vi "EOL_ITECHData.vi"(8 "Exit Program":refnum<vi>, 9 "PS Voltage":dbl=13.5, 10 "idx":u16, 11 "VISA name":refnum<visa-resource-name>) -> ()   [LabVIEW 2018]
uses:
  ZUP_Current/Def Ctrl/TestSeq.ctl
  ZUP_Current/Data buffer/ST0 current buffer.vi
  ZUP_Current/Data buffer/ST1 current buffer.vi
  ZUP_Current/Data buffer/ST2 current buffer.vi
  ZUP_Current/Data buffer/ST3 current buffer.vi
  ZUP_Current/Data buffer/ST4 current buffer.vi
  ZUP_Current/Data buffer/ST5 current buffer.vi
  05.UserVI's/Lambda Power/ITECH/IT-M3100.lvlib
panel:
  in  "Serial Configuration":T1={"Baud Rate"=9600, "Parity"=0, "Data Bits"=8, "Stop Bits"=10} {"Stop Bits" items=["1.0"=10, "1.5"=15, "2.0"=20]; "Data Bits" items=["7"=7, "8"=8]; "Parity" items=["None", "Odd", "Even", "Mark", "Space"]; "Baud Rate" items=["300"=300, "600"=600, "1200"=1200, "2400"=2400, "4800"=4800, "9600"=9600, "19200"=19200]}
  out "Max Cur":dbl
  out "Cur":dbl
  out "loss?":bool
  out "Packet loss":i32
  out "current":dbl(graph)
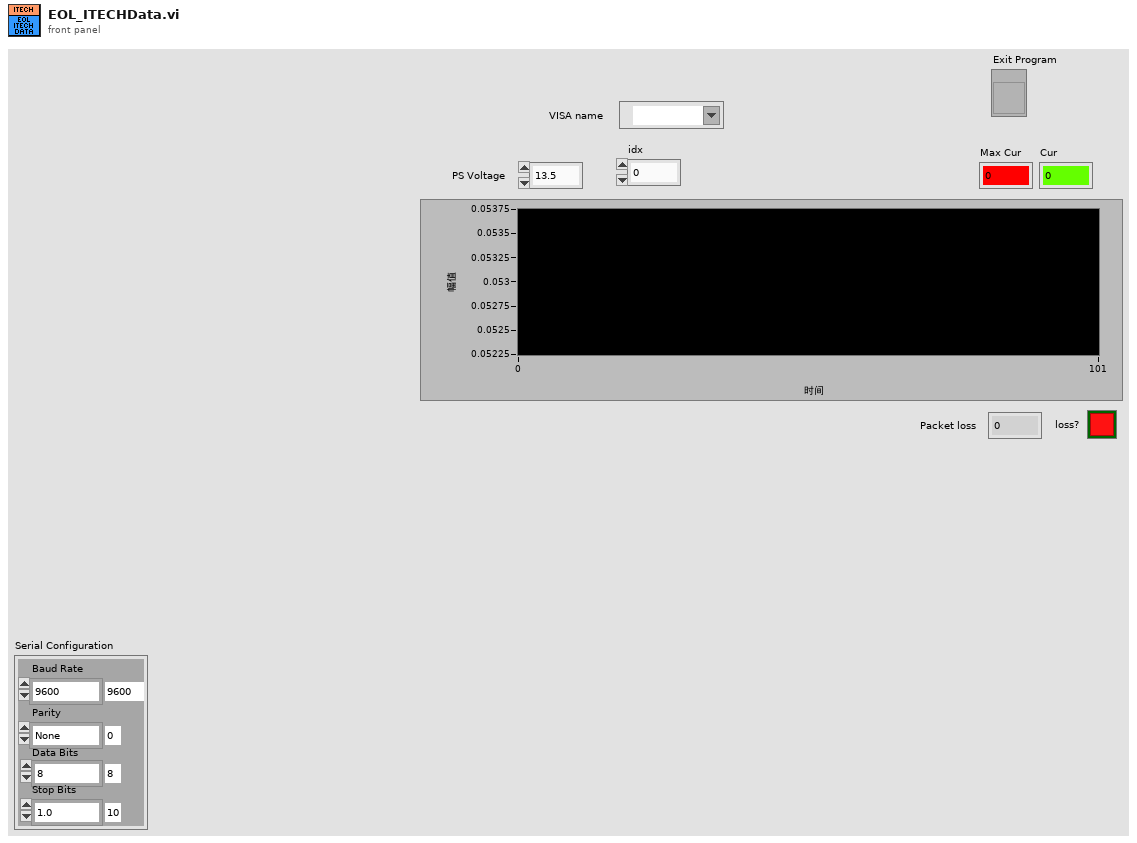
[diagram p1: front panel]
types:
  T1 = cluster{"Baud Rate":u32, "Parity":u16, "Data Bits":u16, "Stop Bits":u16}
  T2 = typedef "TestSeq.ctl" = enum16{"Idle", "Re Connect", "Error", "Initial", "Set Voltage", "Set Current", "Set Out", "Check Voltage", "Check Current", "Check Version No", "Check Out", "Get Current Data", "EOL Get Current Data"}
  T3 = cluster{"Serial Configuration":cluster{"Baud Rate":u32, "Parity":u16, "Data Bits":u16, "Stop Bits":u16}, "VISA name":refnum<visa-resource-name>, "MsgRec":string, "Current buffer":dbl[], "Timer":i32, "CycleNumb":i32, "Error":errorcluster, "Max Cur":dbl, "PS Voltage":dbl}
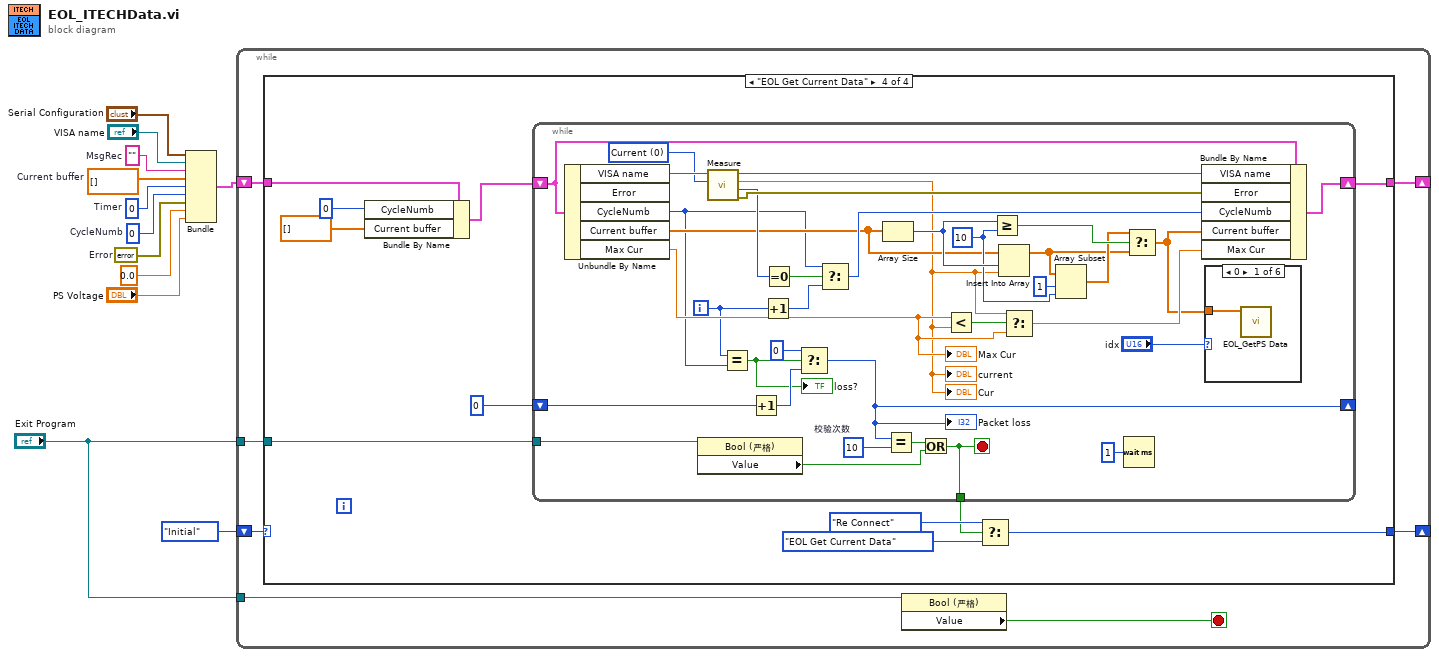
[diagram p0: block diagram]
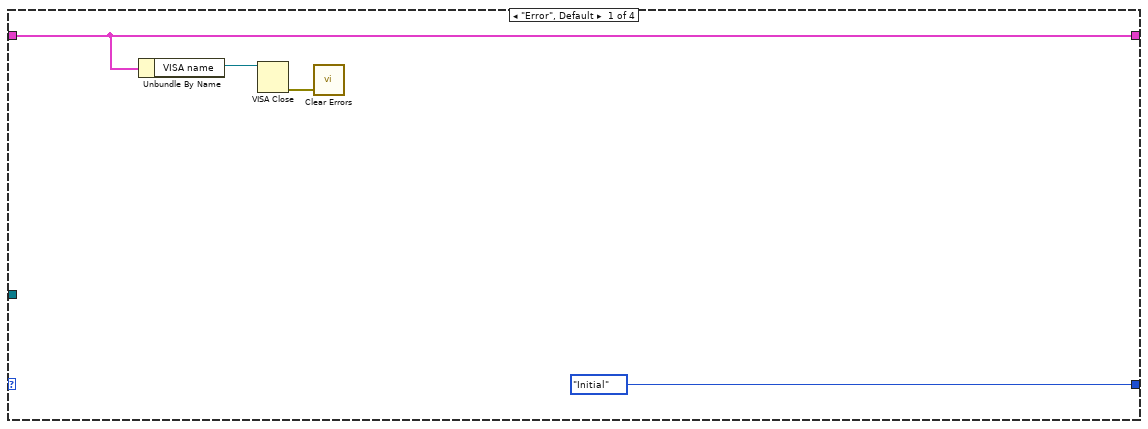
[diagram p2: hidden frame]
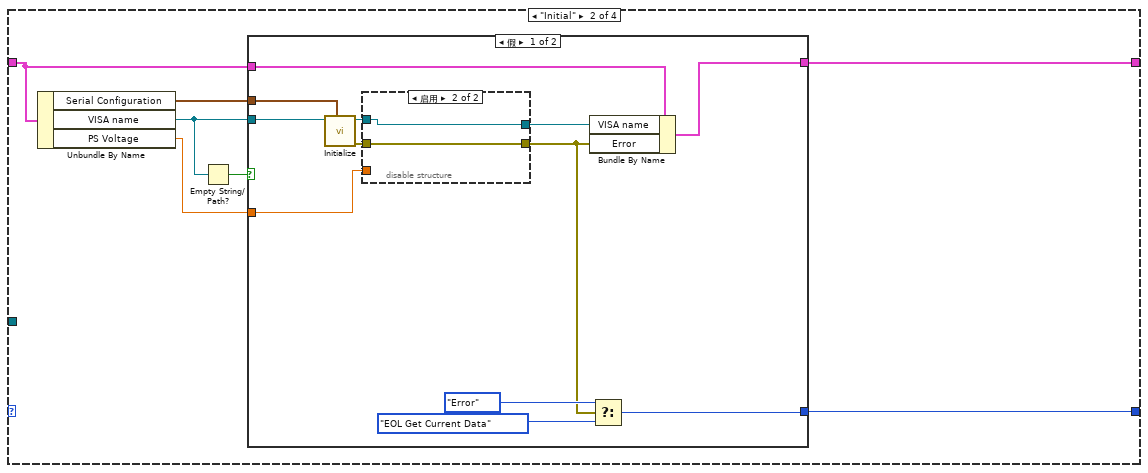
[diagram p3: hidden frame]
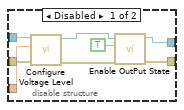
[diagram p4: hidden frame]
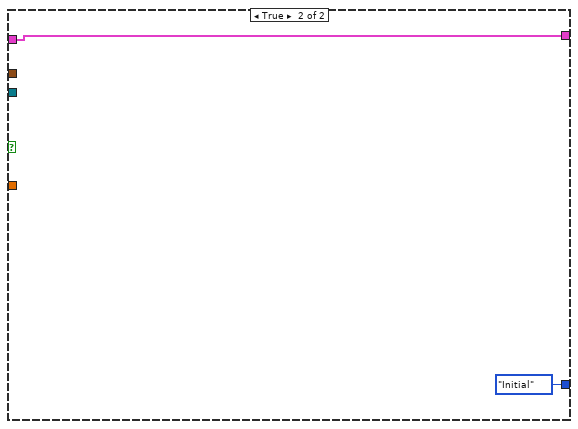
[diagram p5: hidden frame]
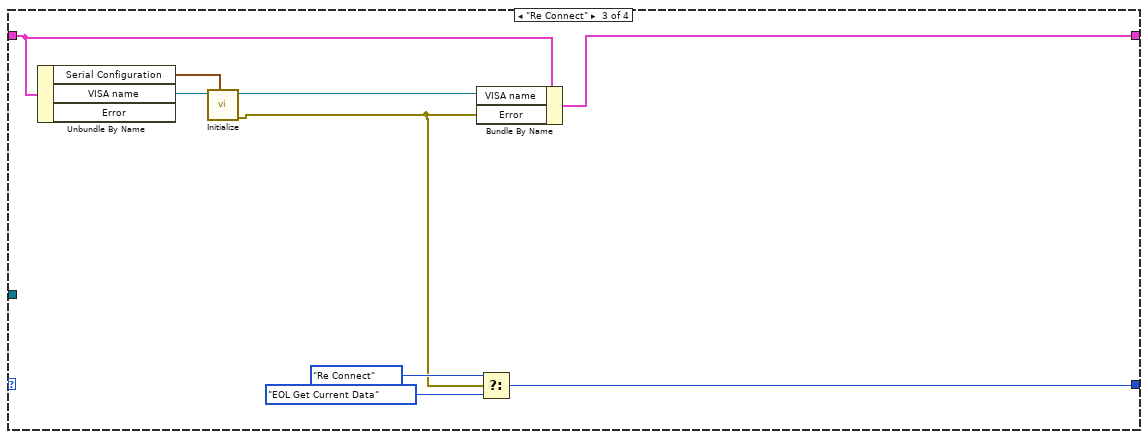
[diagram p6: hidden frame]
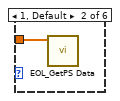
[diagram p7: hidden frame]
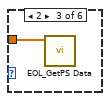
[diagram p8: hidden frame]
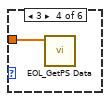
[diagram p9: hidden frame]
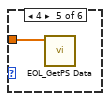
[diagram p10: hidden frame]
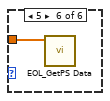
[diagram p11: hidden frame]
diagram:
  w5 = errorcluster {"status"=FALSE, "code"=0, "source"=""}  # Error
  w8 = 0  # CycleNumb
  w9 = 0  # Timer
  w12 = ""  # MsgRec
  w11 = dbl[] []  # Current buffer
  n1 = Bundle("Serial Configuration"="Serial Configuration", "VISA name"="VISA name", "MsgRec"=w12, "Current buffer"=w11, "Timer"=w9, "CycleNumb"=w8, "Error"=w5, "Max Cur"=0.0, "PS Voltage"="PS Voltage") -> (w7:T3)  [unwired: 1 in]
  n2 = while {
    shift-right: [w17] -> _
    shift-left: w7 -> [w18]
    shift-right: [w16] -> _
    shift-left: TestSeq."Initial" -> [w19]
    tunnel: "Exit Program" -> [w14]
    tunnel: "Exit Program" -> [w13]
    stop <- w15 stop-if-true
    n3 = case shown="\"EOL Get Current Data\"" w19 {
      tunnel: w18 -> [w21 w30 w63 w70]
      tunnel: [w21 w29 w62 w73] -> w17
      tunnel: [TestSeq."Initial" w28 w60 w67] -> w16
      tunnel: w13 -> [_ _ _ w65]
      frame "Error", Default {
        n4 = Unbundle By Name(w21) -> ("VISA name"=w22:refnum<visa-resource-name>)
        n5 = VISA Close(VISA resource name=w22) -> (error out=w20:errorcluster)  [unwired: 1 in]
        n6 = call <vilib>:"Clear Errors.vi"("error in (no error)"=w20) -> ()  [unwired: 5 in, 2 out]
      }
      frame "Initial" {
        n7 = Unbundle By Name(w30) -> ("Serial Configuration"=w27:T1, "VISA name"=w26:refnum<visa-resource-name>, "PS Voltage"=w24:dbl)
        n8 = Empty String/Path?(string/path=w26) -> (empty?=w25:bool)
        n9 = case shown="假" w25 {
          tunnel: w30 -> [w42 w54]
          tunnel: [w41 w54] -> w29
          tunnel: w26 -> [w40 _]
          tunnel: [w38 TestSeq."Initial"] -> w28
          tunnel: w27 -> [w36 _]
          tunnel: w24 -> [w31 _]
          frame False {
            n10 = call "Initialize.vi"("Serial Configuration"=w36, "VISA resource name"=w40) -> ("error out"=w33:errorcluster, "VISA resource name out"=w32:refnum<visa-resource-name>)  [unwired: 8 in]
            n11 = disable-structure shown="启用" {
              disable-tunnel: [w50 w51] -> w35
              disable-tunnel: [w49 w52] -> w34
              disable-tunnel: w33 -> [w47 w51]
              disable-tunnel: w32 -> [w45 w52]
              disable-tunnel: w31 -> [w43 _]
              frame Disabled {
                n12 = call "Configure Voltage Level.vi"("error in"=w47, "Level(V)"=w43, "VISA resource name"=w45) -> ("error out"=w46:errorcluster, "VISA resource name out"=w44:refnum<visa-resource-name>)  [unwired: 7 in]
                n13 = call "Enable OutPut State.vi"("error in"=w46, "State"=TRUE, "VISA resource name"=w44) -> ("error out"=w50:errorcluster, "VISA resource name out"=w49:refnum<visa-resource-name>)  [unwired: 7 in]
              }
              frame Enabled {
              }
            }
            n14 = Bundle By Name(cluster=w42, "VISA name"=w34, "Error"=w35) -> (w41:T3)
            n15 = Select(t=TestSeq."Error", s=w35, f=TestSeq."EOL Get Current Data") -> (s? t:f=w38:T2)
          }
          frame True {
          }
        }
      }
      frame "Re Connect" {
        n16 = Unbundle By Name(w63) -> ("Serial Configuration"=w57:T1, "VISA name"=w58:refnum<visa-resource-name>)  [unwired: 1 out]
        n17 = call "Initialize.vi"("Serial Configuration"=w57, "VISA resource name"=w58) -> ("error out"=w55:errorcluster, "VISA resource name out"=w56:refnum<visa-resource-name>)  [unwired: 8 in]
        n18 = Bundle By Name(cluster=w63, "VISA name"=w56, "Error"=w55) -> (w62:T3)
        n19 = Select(t=TestSeq."Re Connect", s=w55, f=TestSeq."EOL Get Current Data") -> (s? t:f=w60:T2)
      }
      frame "EOL Get Current Data" {
        n20 = Bundle By Name(cluster=w70, "CycleNumb"=0, "Current buffer"=dbl[] []) -> (w69:T3)
        n21 = while {
          shift-right: [w107] -> w73
          shift-left: w69 -> [w108]
          shift-right: [w81] -> _
          shift-left: 0 -> [w100]
          tunnel: w65 -> [w96]
          tunnel: [w79] -> w64
          i -> [w78]
          stop <- w79 stop-if-true
          w92 = 10 ("y")
          w98 = u32 10  # 校验次数
          w109 = 0 items=["Current", "Power", "Voltage", "Capacity"] ("Measure Type")
          n22 = Unbundle By Name(w108) -> ("VISA name"=w110:refnum<visa-resource-name>, "CycleNumb"=w77:i32, "Current buffer"=w90:dbl[], "Max Cur"=w83:dbl)  [unwired: 1 out]
          "Max Cur" <- w83
          n23 = property class="Bool (严格)"(reference=w96) -> ("Value"=w95:bool)  [unwired: 1 in, 2 out]
          n24 = call "Measure.vi"("Measure Type"=w109, "VISA resource name"=w110) -> ("error out"=w105:errorcluster, "返回数"=w104:u32, "Value"=w76:dbl, "VISA resource name out"=w106:refnum<visa-resource-name>)  [unwired: 6 in]
          "current" <- w76
          "Cur" <- w76
          n25 = Equal?(x=w78, y=w77) -> (x = y?=w82:bool)
          "loss?" <- w82
          n26 = Increment(x=w100) -> (x+1=w99:u32)
          n27 = Increment(x=w78) -> (x+1=w80:i32)
          n28 = Equal To 0?(x=w104) -> (x = 0?=w103:bool)
          n29 = Select(t=u32 0, s=w82, f=w99) -> (s? t:f=w81:u32)
          "Packet loss" <- w81
          n30 = Select(t=w77, s=w103, f=w80) -> (s? t:f=w102:i32)
          n31 = Array Size(array=w90) -> (size(s)=w94:i32)
          n32 = Equal?(x=w81, y=w98) -> (x = y?=w97:bool)
          n33 = Or(x=w97, y=w95) -> (x .or. y?=w79:bool)
          n34 = Less?(x=w83, y=w76) -> (x < y?=w91:bool)
          n35 = Greater Or Equal?(x=w94, y=w92) -> (x >= y?=w89:bool)
          n36 = Insert Into Array(array=w90, index=w94, new element=w76) -> (w87:dbl[])
          n37 = Select(t=w76, s=w91, f=w83) -> (s? t:f=w86:dbl)
          n38 = Array Subset(array=w87, index=1 ("索引"), length=w92) -> (w88:dbl[])
          n39 = Wait (ms)(milliseconds to wait=u32 1 ("等待时间（毫秒）")) -> ()  [unwired: 1 out]
          n40 = Select(t=w88, s=w89, f=w87) -> (s? t:f=w85:dbl[])
          n41 = Bundle By Name(cluster=w108, "VISA name"=w106, "Error"=w105, "CycleNumb"=w102, "Current buffer"=w85, "Max Cur"=w86) -> (w107:T3)
          n42 = case shown="0" "idx" {
            tunnel: w85 -> [w111 w112 w113 w114 w115 w116]
            frame 0 {
              n43 = call-poly "EOL_GetPS Data.vi"("in"=w111) -> ()  [unwired: 9 in, 2 out]
            }
            frame 1, Default {
              n44 = call-poly "EOL_GetPS Data.vi"("in"=w112) -> ()  [unwired: 9 in, 2 out]
            }
            frame 2 {
              n45 = call-poly "EOL_GetPS Data.vi"("in"=w113) -> ()  [unwired: 9 in, 2 out]
            }
            frame 3 {
              n46 = call-poly "EOL_GetPS Data.vi"("in"=w114) -> ()  [unwired: 9 in, 2 out]
            }
            frame 4 {
              n47 = call-poly "EOL_GetPS Data.vi"("in"=w115) -> ()  [unwired: 9 in, 2 out]
            }
            frame 5 {
              n48 = call-poly "EOL_GetPS Data.vi"("in"=w116) -> ()  [unwired: 9 in, 2 out]
            }
          }
        }
        n49 = Select(t=TestSeq."Re Connect", s=w64, f=TestSeq."EOL Get Current Data") -> (s? t:f=w67:T2)
      }
    }
    n50 = property class="Bool (严格)"(reference=w14) -> ("Value"=w15:bool)  [unwired: 1 in, 2 out]
  }
